vi "Datalog_Read.vi"() -> ()   [LabVIEW 2023]
panel:
  out "record(s)":cluster{"이름":string, "학번":string, "점수":dbl}[](array[cluster])
  in  "datalog path (use dialog)":path
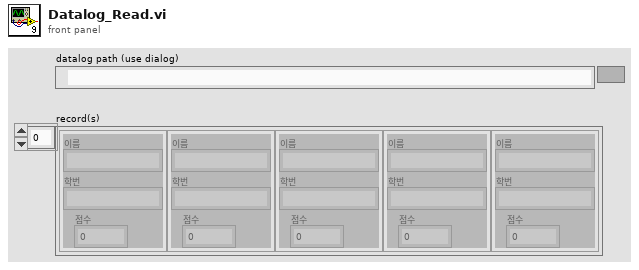
[diagram p1: front panel]
types:
  T1 = enum16{"open", "replace", "create", "open or create", "replace or create", "replace or create with confirmation"}
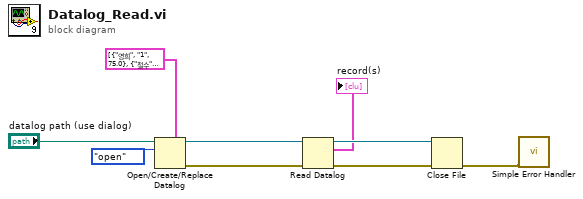
[diagram p0: block diagram]
diagram:
  n1 = Open/Create/Replace Datalog(5:cluster{"이름":string, "학번":string, "점수":dbl}[] [{"이름"="영희", "학번"="1", "점수"=75.0}, {"이름"="철수", "학번"="2", "점수"=83.0}, {"이름"="홍길동", "학번"="3", "점수"=66.0}] ("병아리반 영어점수"), 10:T1."open" ("operation (0:open)"), 11:"datalog path (use dialog)") -> (0:w9:errorcluster, 3:w6:refnum<k1>)  [unwired: 3 in, 1 out]
  n2 = Read Datalog(4:w9, 7:w6) -> (0:w8:errorcluster, 2:→"record(s)":cluster{"이름":string, "학번":string, "점수":dbl}[], 3:w5:refnum<k1>)  [unwired: 1 in]
  n3 = Close File(refnum=w5, error in=w8) -> (error out=w2:errorcluster)  [unwired: 1 out]
  n4 = call <vilib>:"Simple Error Handler.vi"("error in (no error)"=w2) -> ()  [unwired: 4 in, 5 out]
